vi "repPrepareFreeBallPlayVSS.vi"(8 "error in (no error)":errorcluster, 9 "Game in 2":refnum<class "Game.lvclass">, 10 "RobotPlacement":T1(array[cluster]), 11 "PrepareFreeBallPlayVSS in":refnum<class "PrepareFreeBallPlayVSS.lvclass">) -> (0 "error out":errorcluster, 2 "RobotPlacement 2":T1(array[cluster]), 3 "PrepareFreeBallPlayVSS out":refnum<class "PrepareFreeBallPlayVSS.lvclass">)   [LabVIEW 2020, in "PrepareFreeBallPlayVSS.lvclass"]
uses:
  PrepareFreeBallPlayVSS.lvclass
  Game_class/Game.lvclass
  Game_class/Game.lvclass/Game.ctl
  Object_class/Object.lvclass/Object.ctl
  Team_class/Team.lvclass/Team.ctl
  Robot_class/Robot.lvclass/Robot.ctl
  Object_class/Read x.vi
  Object_class/Read y.vi
  Robot_class/Read orientation.vi
  Game_class/Read FieldRef.vi
  Game_class/Read BallRef.vi
  Game_class/Read KeeperTeam.vi
  Team_class/Read RobotRef.vi
  Ally_class/Ally.lvclass
  C:/ROBOIME/SSL_AI/Team_class/Team.lvclass
  Ball_class/Ball.lvclass
  C:/ROBOIME/SSL_AI/Object_class/Object.lvclass
  Robot_class/Robot.lvclass
  Field_class/Field.lvclass
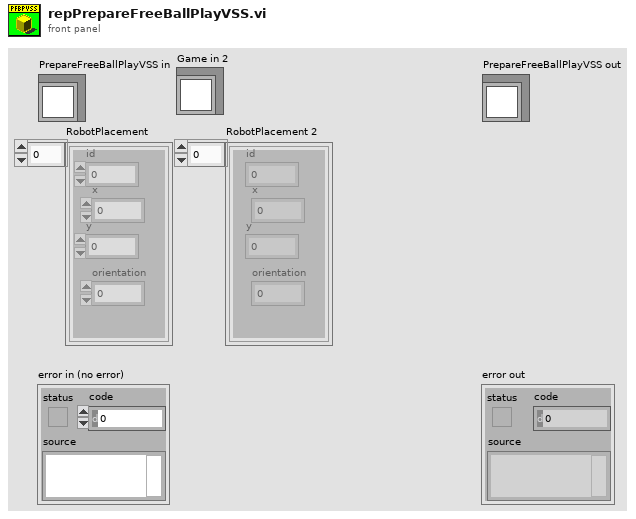
[diagram p1: front panel]
types:
  T1 = cluster{"id":i32, "x":dbl, "y":dbl, "orientation":dbl}[]
  T2 = cluster{"id":i32, "x":dbl, "y":dbl, "orientation":dbl}
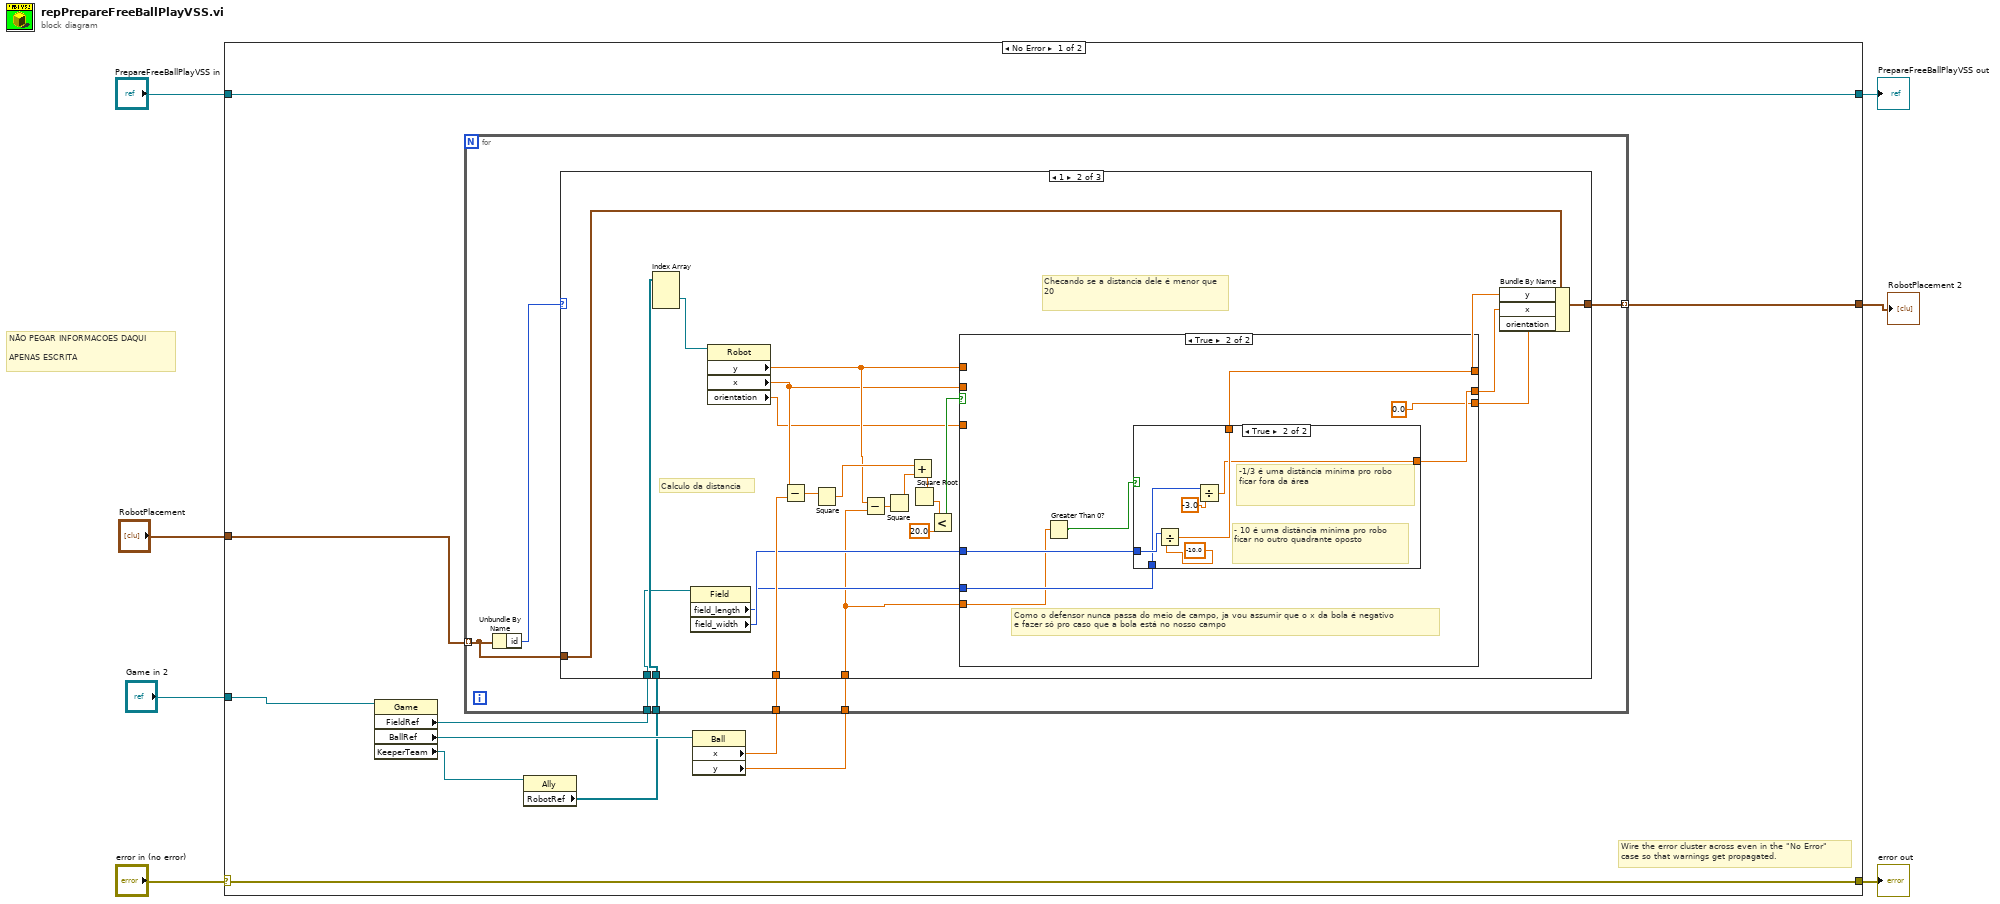
[diagram p0: block diagram]
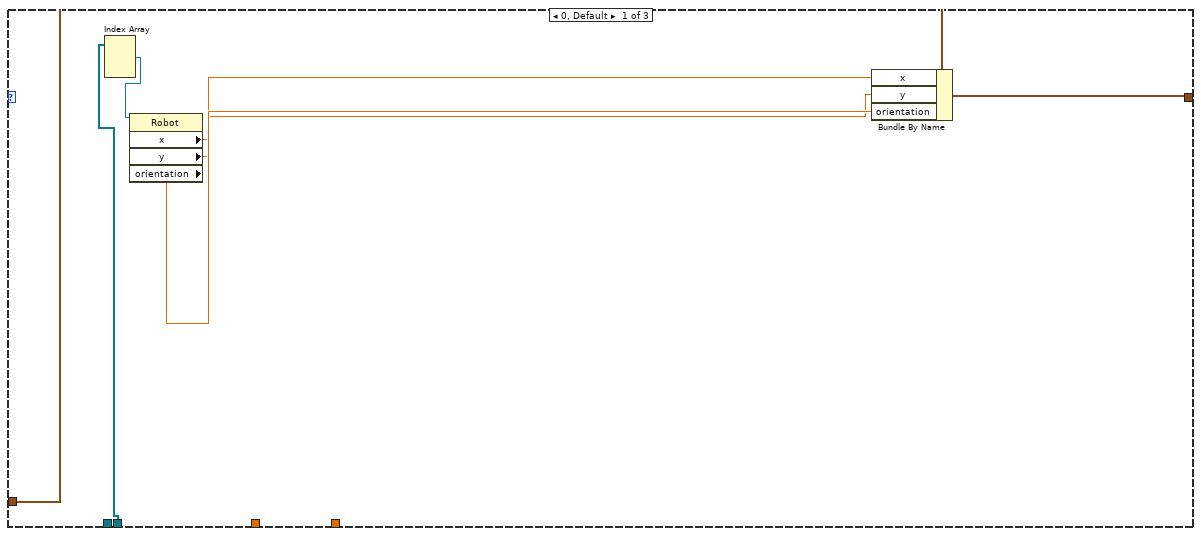
[diagram p2: hidden frame]
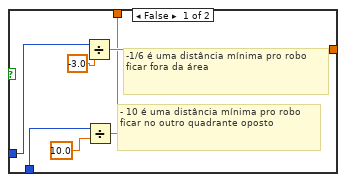
[diagram p4: hidden frame]
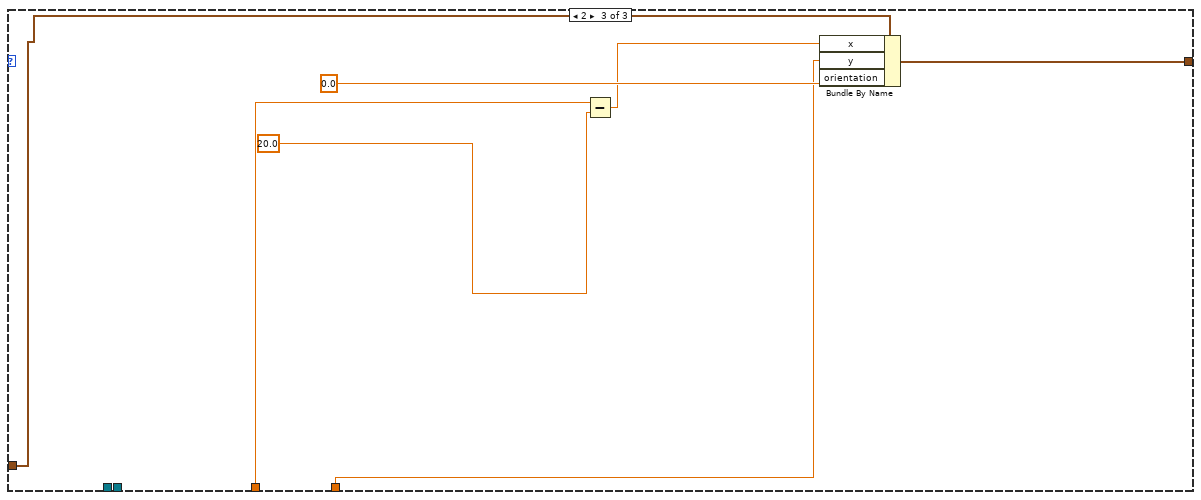
[diagram p5: hidden frame]
diagram:
  # "NÃO PEGAR INFORMACOES DAQUI\n\nAPENAS ESCRITA"
  n1 = case shown="No Error" "error in (no error)" {
    selector: "error in (no error)" -> [w17 w86]
    tunnel: [w17 w86] -> w6
    tunnel: [w18 w85] -> w4
    tunnel: "PrepareFreeBallPlayVSS in" -> [w18 w85]
    tunnel: "RobotPlacement" -> [w15 _]
    tunnel: "Game in 2" -> [w16 _]
    tunnel: [w14 _] -> w1
    frame No Error {
      # "Wire the error cluster across even in the \"No Error\"\ncase so that warnings get propagated."
      n2 = property class="Game"(reference=w16) -> ("FieldRef"=w13:refnum<class "Field.lvclass">, "BallRef"=w12:refnum<class "Ball.lvclass">, "KeeperTeam"=w11:refnum<class "Ally.lvclass">)  [unwired: 1 in, 2 out]
      n3 = property class="Ally"(reference=w11) -> ("RobotRef"=w10:refnum<class "Robot.lvclass">[])  [unwired: 1 in, 2 out]
      n4 = property class="Ball"(reference=w12) -> ("x"=w9:dbl, "y"=w8:dbl)  [unwired: 1 in, 2 out]
      n5 = for {
        tunnel: w15 -> [w24] mode=indexing
        tunnel: [w23] -> w14 mode=indexing
        tunnel: w13 -> [w22]
        tunnel: w10 -> [w21]
        tunnel: w9 -> [w20]
        tunnel: w8 -> [w19]
        n6 = Unbundle By Name(w24) -> ("id"=w25:i32)
        n7 = case shown="1" w25 {
          tunnel: w24 -> [w32 w55 w84]
          tunnel: [w31 w54 w83] -> w23
          tunnel: w22 -> [_ w39 _]
          tunnel: w21 -> [w27 w53 _]
          tunnel: w20 -> [_ w51 w79]
          tunnel: w19 -> [_ w33 w78]
          frame 0, Default {
            n8 = Index Array(array=w27) -> (element #1=w26:refnum<class "Robot.lvclass">)  [unwired: 3 in, 2 out]
            n9 = property class="Robot"(reference=w26) -> ("x"=w28:dbl, "y"=w29:dbl, "orientation"=w30:dbl)  [unwired: 1 in, 2 out]
            n10 = Bundle By Name(cluster=w32, "x"=w28, "y"=w29, "orientation"=w30) -> (w31:T2)
          }
          frame 1 {
            # "Calculo da distancia"
            # "Checando se a distancia dele é menor que 20"
            n11 = Index Array(array=w53) -> (element #2=w52:refnum<class "Robot.lvclass">)  [unwired: 3 in, 2 out]
            n12 = property class="Field"(reference=w39) -> ("field_length"=w37:i32, "field_width"=w38:i32)  [unwired: 1 in, 2 out]
            n13 = property class="Robot"(reference=w52) -> ("y"=w45:dbl, "x"=w43:dbl, "orientation"=w41:dbl)  [unwired: 1 in, 2 out]
            n14 = Subtract(x=w43, y=w51) -> (x-y=w50:dbl)
            n15 = Square(x=w50) -> (x^2=w47:dbl)
            n16 = Subtract(x=w45, y=w33) -> (x-y=w49:dbl)
            n17 = Square(x=w49) -> (x^2=w48:dbl)
            n18 = Add(x=w47, y=w48) -> (x+y=w35:dbl)
            n19 = Square Root(x=w35) -> (sqrt(x)=w36:dbl)
            n20 = Less?(x=w36, y=20.0) -> (x < y?=w46:bool)
            n21 = case shown="True" w46 {
              tunnel: [w58 w64] -> w44
              tunnel: w45 -> [w58 _]
              tunnel: [w57 w61] -> w42
              tunnel: w43 -> [w57 _]
              tunnel: [w56 0.0] -> w40
              tunnel: w41 -> [w56 _]
              tunnel: w38 -> [_ w63]
              tunnel: w37 -> [_ w62]
              tunnel: w33 -> [_ w59]
              frame False {
              }
              frame True {
                # "Como o defensor nunca passa do meio de campo, ja vou assumir que o x da bola é negativo\ne fazer só pro caso que a bola está no nosso campo"
                n22 = Greater Than 0?(x=w59) -> (x > 0?=w65:bool)
                n23 = case shown="True" w65 {
                  tunnel: [w67 w76] -> w64
                  tunnel: w63 -> [w66 w75]
                  tunnel: w62 -> [w69 w72]
                  tunnel: [w68 w73] -> w61
                  frame False {
                    # "- 10 é uma distância mínima pro robo\nficar no outro quadrante oposto"
                    # "-1/6 é uma distância mínima pro robo\nficar fora da área"
                    n24 = Divide(x=w66, y=-3.0) -> (x/y=w68:dbl)
                    n25 = Divide(x=w69, y=10.0) -> (x/y=w67:dbl)
                  }
                  frame True {
                    # "-1/3 é uma distância mínima pro robo\nficar fora da área"
                    # "- 10 é uma distância mínima pro robo\nficar no outro quadrante oposto"
                    n26 = Divide(x=w75, y=-10.0) -> (x/y=w76:dbl)
                    n27 = Divide(x=w72, y=-3.0) -> (x/y=w73:dbl)
                  }
                }
              }
            }
            n28 = Bundle By Name(cluster=w55, "y"=w44, "x"=w42, "orientation"=w40) -> (w54:T2)
          }
          frame 2 {
            n29 = Subtract(x=w79, y=20.0 ("x")) -> (x-y=w80:dbl)
            n30 = Bundle By Name(cluster=w84, "x"=w80, "y"=w78, "orientation"=0.0) -> (w83:T2)
          }
        }
      }
    }
    frame Error {
    }
  }
  "error out" <- w6
  "PrepareFreeBallPlayVSS out" <- w4
  "RobotPlacement 2" <- w1
